vi "FilterResults.vi"(8 "error in (no error)":errorcluster, 11 "CDependencyInspection in":refnum<class "CDependencyInspection.lvclass">) -> (0 "error out":errorcluster, 3 "CDependencyInspection out":refnum<class "CDependencyInspection.lvclass">)   [LabVIEW 2020, in "DependencyInspection.lvlib" / "CDependencyInspection.lvclass"]
uses:
  CDependencyInspection.lvclass
  CDependencyInspection.lvclass/CDependencyInspection.ctl
  CDependencyList/CDependencyList.lvclass
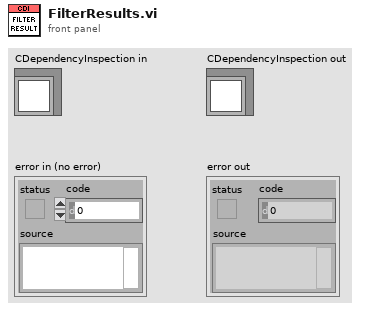
[diagram p1: front panel]
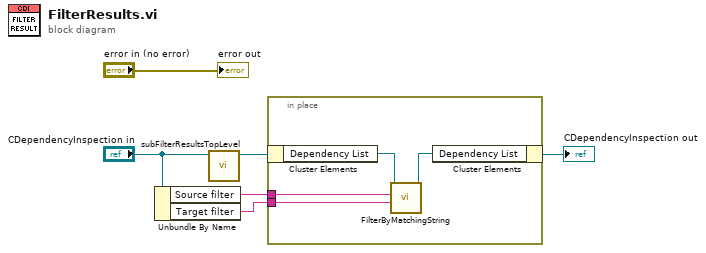
[diagram p0: block diagram]
diagram:
  n1 = Unbundle By Name("CDependencyInspection in") -> ("Source filter"=w2:string, "Target filter"=w1:string)
  n2 = call "subFilterResultsTopLevel.vi"("CDependencyInspection in"="CDependencyInspection in") -> ("CDependencyInspection out"=w5:refnum<class "CDependencyInspection.lvclass">)  [unwired: 9 in, 1 out]
  n3 = in-place {
    in-place-border: w2 -> [w8]
    in-place-border: w1 -> [w7]
    n4 = in-place-cluster #1(w5) -> ("Dependency List"=w10:refnum<class "CDependencyList.lvclass">)
    n5 = call-dynamic "FilterByMatchingString.vi"("Target filter"=w7, "Source filter"=w8, "CDependencyList in"=w10) -> ("CDependencyList out"=w9:refnum<class "CDependencyList.lvclass">)  [unwired: 7 in, 1 out]
    n6 = in-place-cluster #1("Dependency List"=w9) -> (→"CDependencyInspection out":refnum<class "CDependencyInspection.lvclass">)
  }
  "error out" <- "error in (no error)"
